vi "平台远程升级.vi"(8 "error in (no error)":errorcluster) -> (0 "error out":errorcluster)   [LabVIEW 2016, in "数据传输系统-02.lvlib" / "update.lvlib" / "http client.lvclass"]
uses:
  http client.lvclass
  update.lvlib
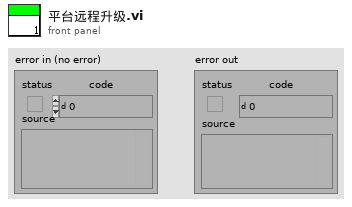
[diagram p1: front panel]
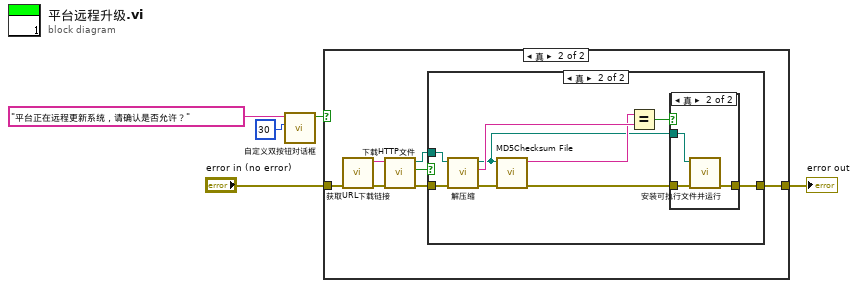
[diagram p0: block diagram]
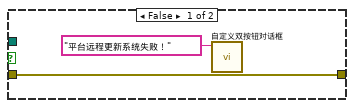
[diagram p3: hidden frame]
diagram:
  n1 = call "自定义双按钮对话框.vi"("数值"=30, "消息"="平台正在远程更新系统，请确认是否允许？") -> ("输出"=w3:bool)  [unwired: 9 in]
  n2 = case shown="真" w3 {
    tunnel: "error in (no error)" -> [w6 w8]
    tunnel: [w6 w7] -> w1
    frame False {
    }
    frame True {
      n3 = call "获取URL下载链接.vi"("error in (no error)"=w8) -> ("error out"=w11:errorcluster, "String/Binary data"=w10:string)  [unwired: 9 in]
      n4 = call "下载HTTP文件.vi"("error in (no error)"=w11, "Base URL"=w10) -> ("error out"=w12:errorcluster, "ok?"=w9:bool, "路径"=w13:path)  [unwired: 7 in]
      n5 = case shown="真" w9 {
        tunnel: w13 -> [_ w24]
        tunnel: w12 -> [w14 w23]
        tunnel: [w14 w16] -> w7
        frame False {
          n6 = call "自定义双按钮对话框.vi"("消息"="平台远程更新系统失败！") -> ()  [unwired: 10 in, 1 out]
        }
        frame True {
          n7 = call "解压缩.vi"("error in (no error)"=w23, "Zip file"=w24) -> ("error out"=w20:errorcluster, "MD5"=w22:string, "待校验的文件路径"=w19:path)  [unwired: 7 in]
          n8 = call <vilib>:"MD5Checksum File.vi"("error in (no error)"=w20, "Path"=w19) -> ("error out"=w18:errorcluster, "MD5 message-digest"=w21:string)  [unwired: 8 in]
          n9 = Equal?(x=w21, y=w22) -> (x = y?=w17:bool)
          n10 = case shown="真" w17 {
            tunnel: w19 -> [_ w28]
            tunnel: w18 -> [w25 w27]
            tunnel: [w25 w26] -> w16
            frame False {
            }
            frame True {
              n11 = call "安装可执行文件并运行.vi"("error in (no error)"=w27, "源路径"=w28) -> ("error out"=w26:errorcluster)  [unwired: 9 in]
            }
          }
        }
      }
    }
  }
  "error out" <- w1
